vi "Concatenate_Blocks.vi"() -> (5 "Plug in titles":string[](array[string]), 7 "Plug in values":string[](array[string]))   [LabVIEW 2012]
uses:
  Controls/Post_Process.ctl
  Controls/Graph_Type.ctl
  Globals/Meas_global.vi
  <vilib>/Analysis/NI_AALBase.lvlib
panel:
  in  "PDF":bool=TRUE
  out "No Of Spectral Averages":i32
  out "Autocorrelation":cluster{dbl, dbl, dbl[]}[](graph)
  in  "Show Smooth":bool=TRUE
  in  "Save Plots":bool
  in  "No of averged samples in spectra":i32=4096
  in  "Calculate Spectra and Histogram?":bool
  out "Spectra":cluster{dbl, dbl, dbl[]}[](graph)
  in  "Averaging samples":i32=5 min=1 max=1000
  out "Histogram/Pdf":T1(graph)
  out "Waveform Graph":dbl[][](graph)
  in  "Channels to Plot":i32[](array[ring])=[0] items=["FF (C)", "Save Nothing"]
  # "Run this VI to update the channel names"
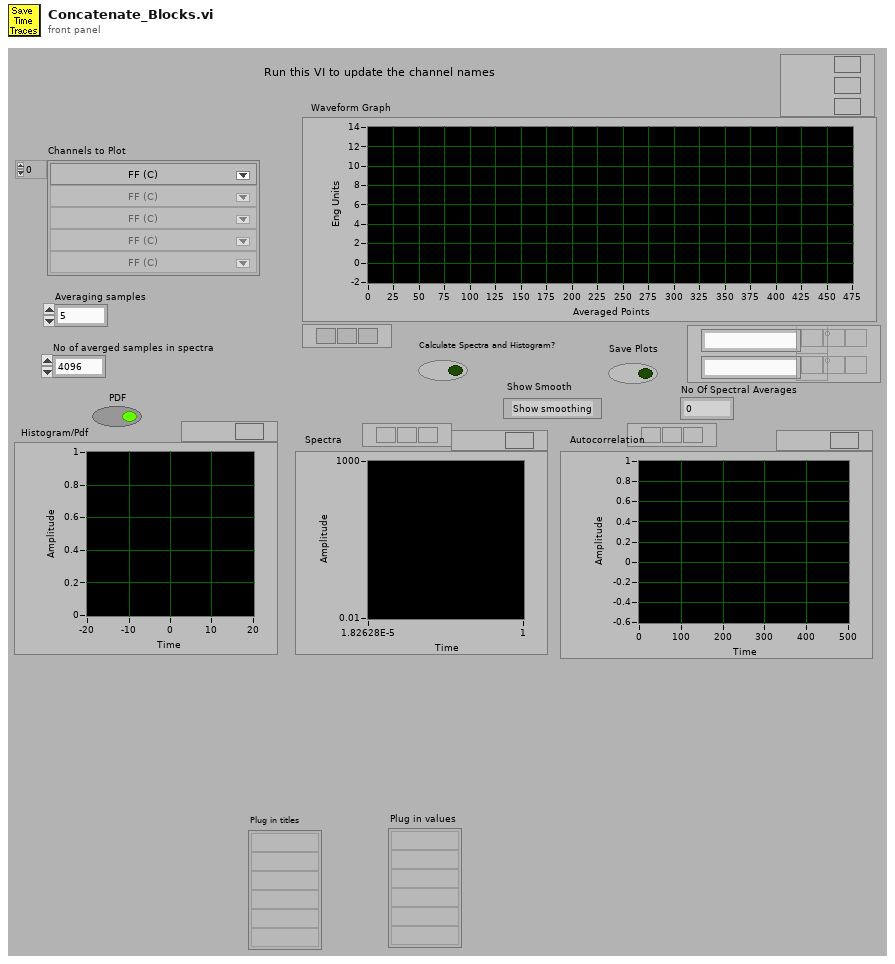
[diagram p1: front panel]
types:
  T1 = cluster{"element":dbl, dbl, "1D histogram or PDF":dbl[]}[]
  T2 = typedef "Analysis_info_cluster.ctl" = cluster{"Colour":u32, "Inst type":T3, "Inst name":string, "Symbol":string, "Code name":string, "Extra Info":string, "Inst Array":T4, "Extra Titles":string[], "Extra Values":string[], "U":dbl, "u^2":dbl, "u^3":dbl, "u^4":dbl, "Skew_u":dbl, "Kurt_u":dbl, "Sd Error in Mean":dbl, "% u'/U":dbl, "X":dbl, "Y":dbl, "Z":dbl, "Timescale integral to 25%":dbl, "Sd Error in Variance":dbl, "Calib File":path, "Calib Constants":dbl[], "Output Position":bool, "Full Stats":bool, "Av Sampling Rate":dbl, "Av No of Samples":dbl, "Total Meas Time (s)":dbl, "ADAM Ch Name":string}
  T3 = typedef "Inst_type.ctl" = enum16{"Propeller anemometer", "Raw voltage", "Pressure Transducer", "Pitot-static tube", "Preston tube", "Hot wire", "Cross wire 1", "Cross wire 2", "Generic Linear", "Generic Polynomial", "Generic BackPoly", "Fast FID", "Thermocouple", "Cold wire", "Pulsed Wire", "LDA Vel", "LDA Tran time", "LDA Arr time"}
  T4 = typedef "Instrument_Array.ctl" = enum16{"PWA", "LDA", "Analogue"}
  T5 = typedef "Time_Trace_Cluster.ctl" = cluster{"Weighting":dbl[], "Time (s)":dbl[], "Voltage":dbl[], "Eng Values":dbl[]}
  T6 = typedef "Post_Process.ctl" = enum16{"Take New Data", "Post Process Raw Data File"}
  T7 = typedef "Graph_Type.ctl" = enum16{"Show no graph", "Voltage trace", "Velocity trace", "Vel histogram", "Spectrum", "f.E(f) v Log f", "Auto-Corr"}
  T8 = cluster{"Plot 1":u16, "Plot 2":u16, "Save graph":u16, "Plot Type":T7}
  T9 = cluster{"element":dbl, dbl, "1D histogram or PDF":dbl[]}
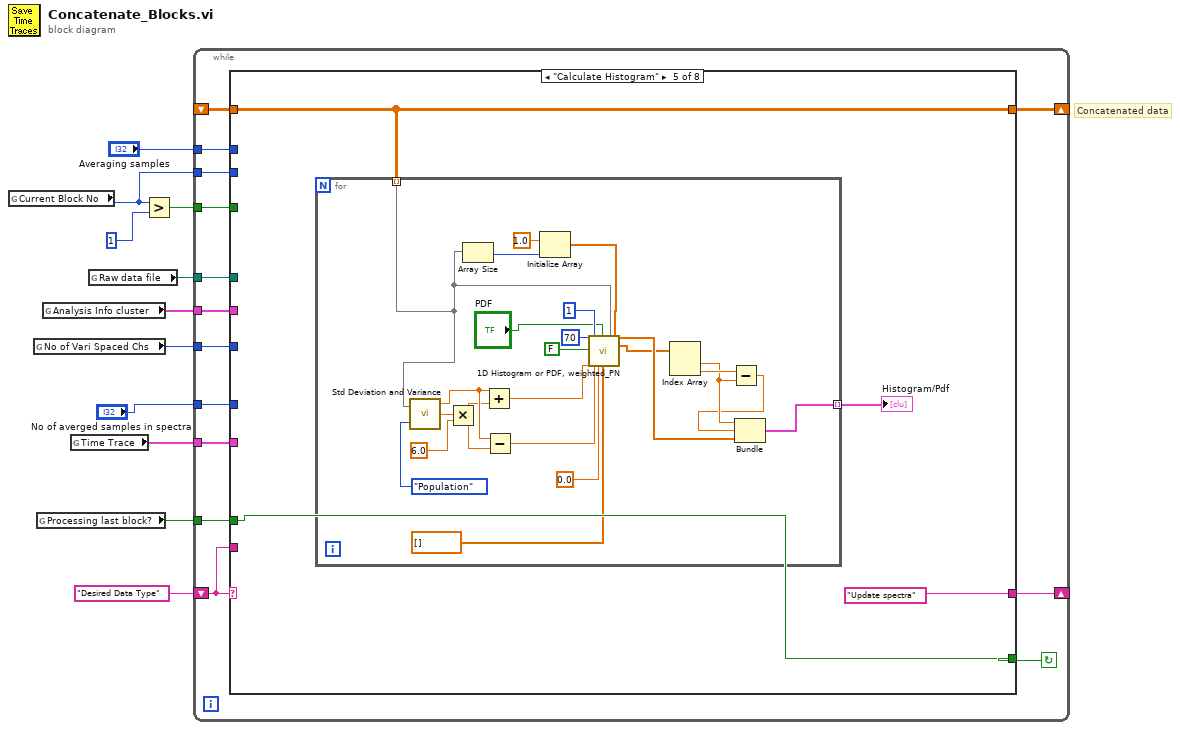
[diagram p0: block diagram]
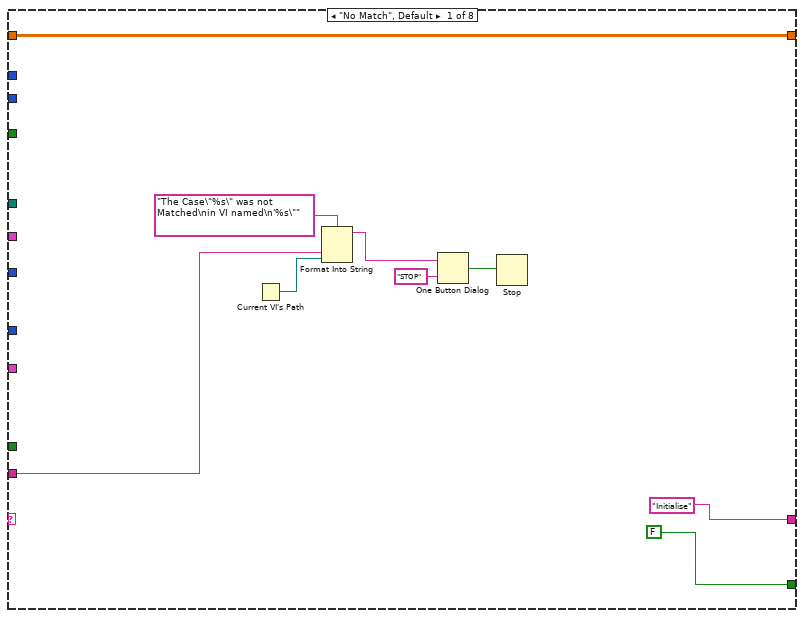
[diagram p2: hidden frame]
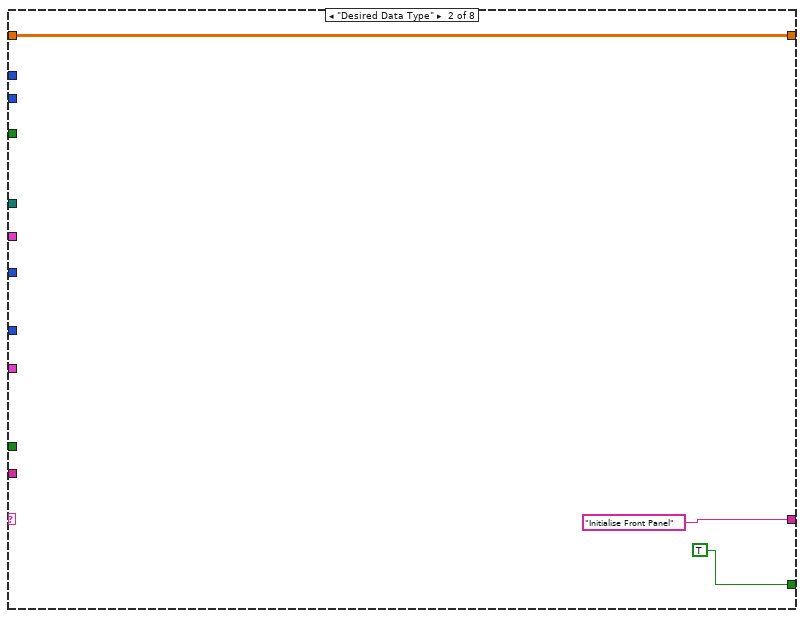
[diagram p3: hidden frame]
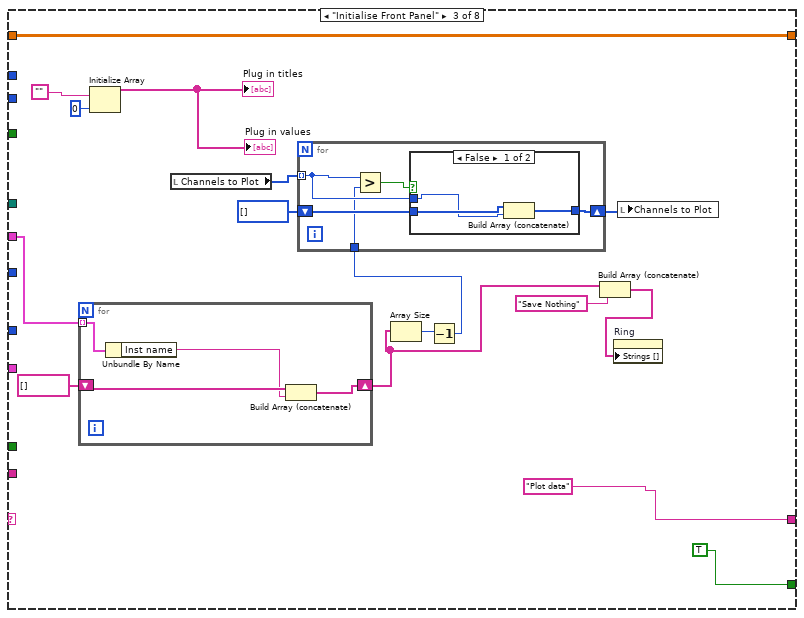
[diagram p4: hidden frame]
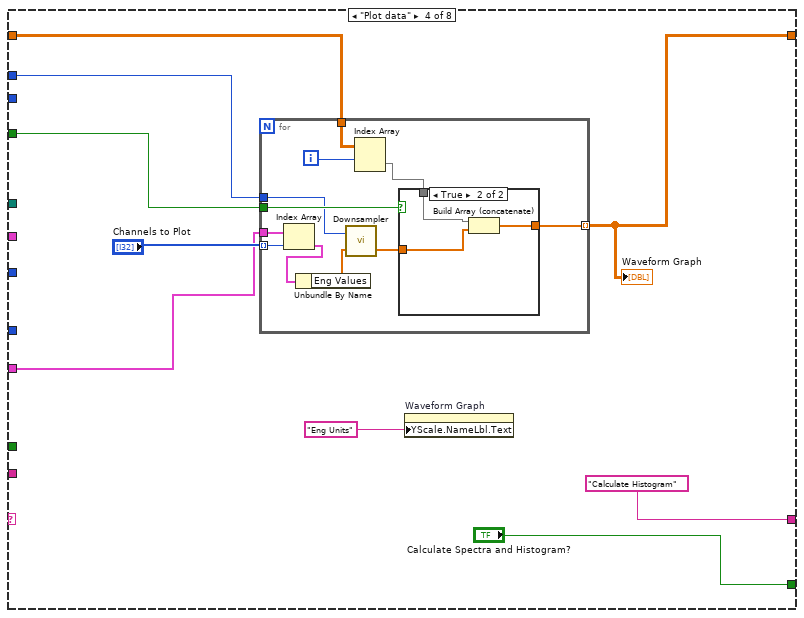
[diagram p6: hidden frame]
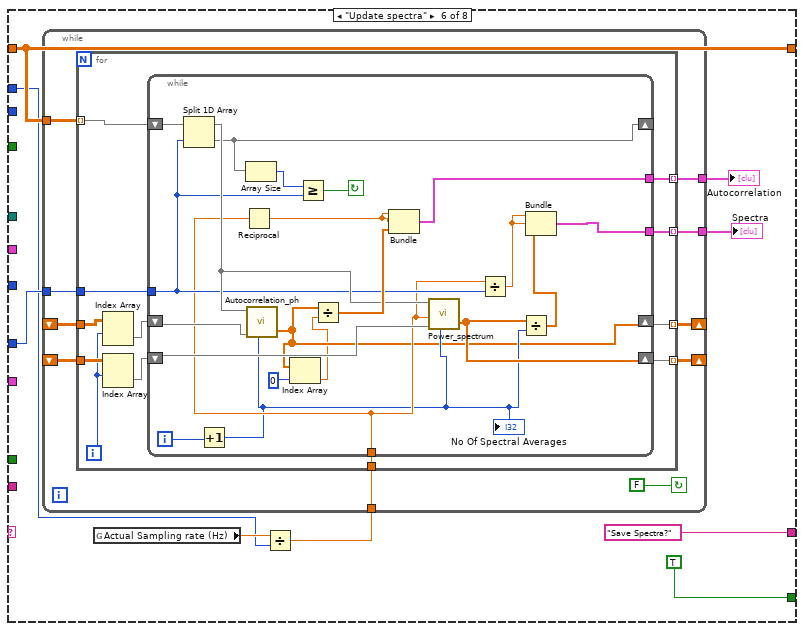
[diagram p8: hidden frame]
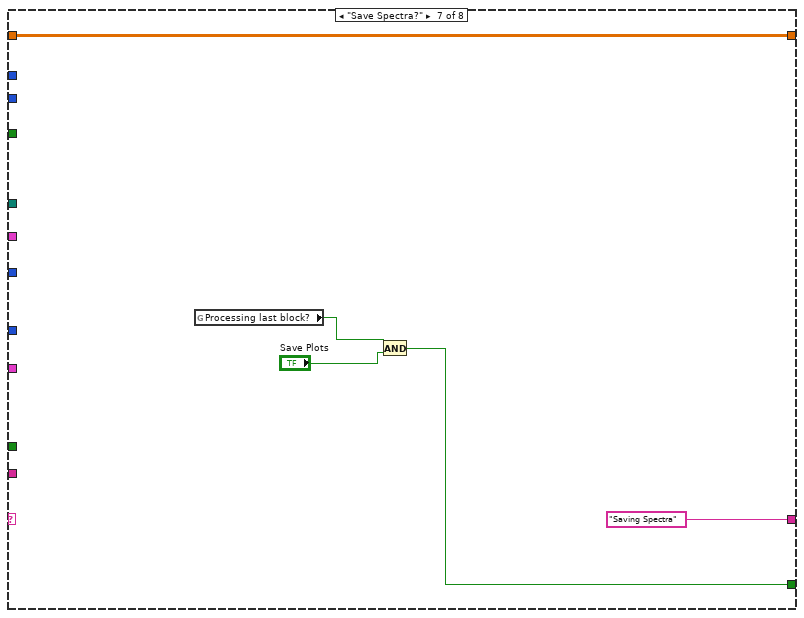
[diagram p9: hidden frame]
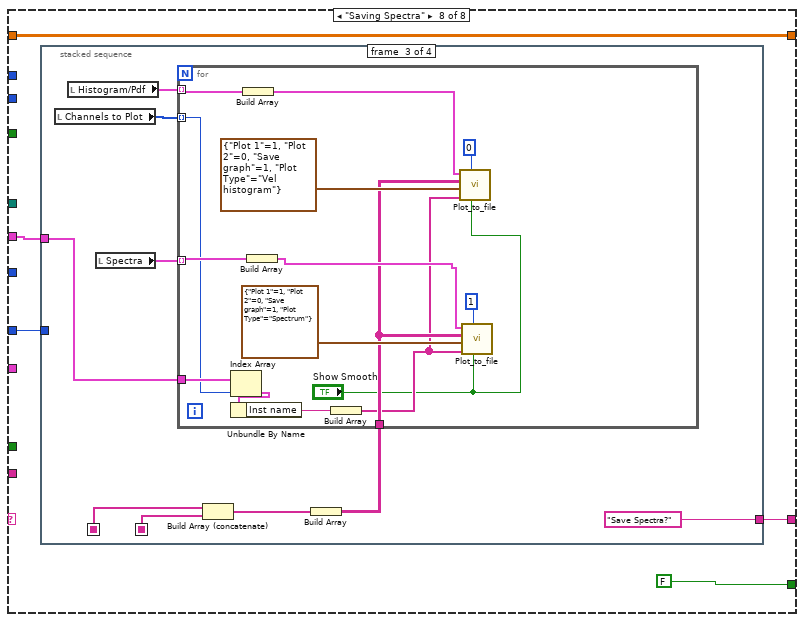
[diagram p10: hidden frame]
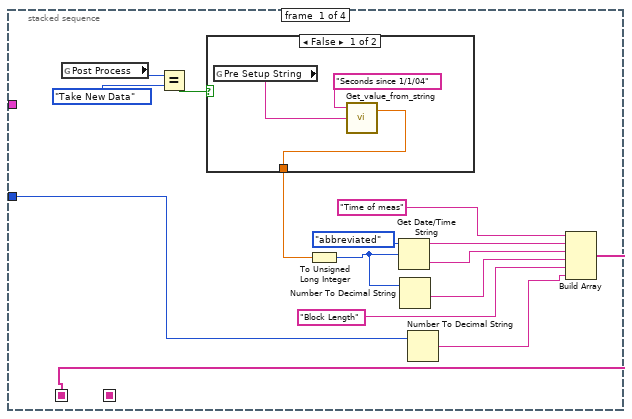
[diagram p11: hidden frame]
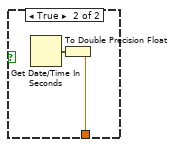
[diagram p12: hidden frame]
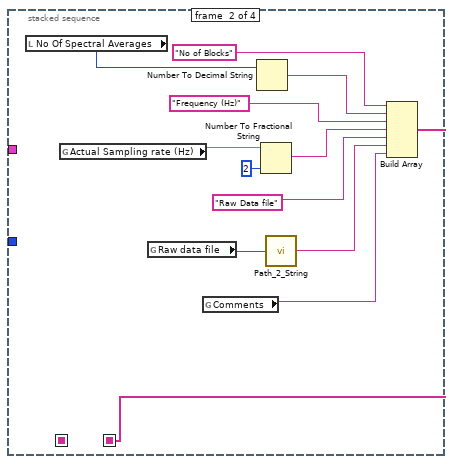
[diagram p13: hidden frame]
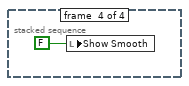
[diagram p14: hidden frame]
diagram:
  # "Concatenated data"
  n1 = global read "Meas_global.vi" "Current Block No"() -> (w8:i32)
  n2 = global read "Meas_global.vi" "No of Vari Spaced Chs"() -> (w6:i32)
  n3 = global read "Meas_global.vi" "Processing last block?"() -> (w1:bool)
  n4 = global read "Meas_global.vi" "Analysis Info cluster"() -> (w7:T2[])
  n5 = global read "Meas_global.vi" "Time Trace"() -> (w3:T5[])
  n6 = global read "Meas_global.vi" "Raw data file"() -> (w10:path)
  n7 = Greater?(x=w8, y=1) -> (0:w5:bool)
  n8 = while {
    shift-left: "Desired Data Type" -> [w23]
    shift-right: [w24] -> _
    tunnel: w10 -> [w22]
    tunnel: w5 -> [w21]
    tunnel: w8 -> [w20]
    tunnel: w7 -> [w19]
    tunnel: w6 -> [w18]
    shift-right: [w16] -> _
    shift-left: _ -> [w17]
    tunnel: "No of averged samples in spectra" -> [w15]
    tunnel: w3 -> [w14]
    tunnel: "Averaging samples" -> [w13]
    tunnel: w1 -> [w12]
    stop <- w25 continue-if-true
    n9 = case shown="\"Calculate Histogram\"" w23 {
      tunnel: [FALSE TRUE TRUE "Calculate Spectra and Histogram?" w92 TRUE ("Calculate Spectra and Histogram?") w170 FALSE ("Calculate Spectra and Histogram?")] -> w25
      tunnel: ["Initialise" "Initialise Front Panel" "Plot data" "Calculate Histogram" ("t") "Update spectra" "Save Spectra?" "Saving Spectra" w178] -> w24
      tunnel: w23 -> [w29 _ _ _ _ _ _ _]
      tunnel: w22 -> [_ _ _ _ _ _ _ _]
      tunnel: w21 -> [_ _ _ w74 _ _ _ _]
      tunnel: w20 -> [_ _ _ _ _ _ _ _]
      tunnel: w19 -> [_ _ w40 _ _ _ _ w177]
      tunnel: w18 -> [_ _ _ _ _ _ _ _]
      tunnel: w17 -> [w26 w35 w43 w75 w94 w123 w174 w179]
      tunnel: [w26 w35 w43 w72 w94 w123 w174 w179] -> w16
      tunnel: w15 -> [_ _ _ _ _ w124 _ w175]
      tunnel: w14 -> [_ _ _ w68 _ _ _ _]
      tunnel: w13 -> [_ _ _ w67 _ w121 _ _]
      tunnel: w12 -> [_ _ _ _ w92 _ _ _]
      frame "No Match", Default {
        n10 = Current VI's Path() -> (path=w28:path)
        n11 = Format Into String(format string="The Case\"%s\" was not Matched\nin VI named\n'%s\"" ("Format String"), w29, w28) -> (resulting string=w32:string)  [unwired: 2 in, 1 out]
        n12 = One Button Dialog(message=w32, button name ("OK")="STOP") -> (true=w30:bool)
        n13 = Stop(stop? (T)=w30) -> ()
      }
      frame "Desired Data Type" {
      }
      frame "Initialise Front Panel" {
        n14 = for {
          tunnel: w40 -> [w57] mode=indexing
          shift-right: [w55] -> w39
          shift-left: string[] [] -> [w56]
          n15 = Unbundle By Name(w57) -> ("Inst name"=w54:string)
          n16 = Build Array (concatenate)(w56, w54) -> (w55:string[])
        }
        n17 = Initialize Array("", 0) -> (→"Plug in values" →"Plug in titles":string[])
        n18 = local read "Channels to Plot"() -> (w50:i32[])
        n19 = Array Size(array=w39) -> (size(s)=w45:i32)
        n20 = Decrement(x=w45) -> (x-1=w44:i32)
        n21 = for {
          tunnel: w50 -> [w59] mode=indexing
          shift-right: [w60] -> w48
          shift-left: i32[] [] -> [w61]
          tunnel: w44 -> [w58]
          n22 = Greater?(x=w59, y=w58) -> (0:w62:bool)
          n23 = case shown="False" w62 {
            tunnel: w61 -> [w65 w66]
            tunnel: [w64 w66] -> w60
            tunnel: w59 -> [w63 _]
            frame False {
              n24 = Build Array (concatenate)(w65, w63) -> (w64:i32[])
            }
            frame True {
            }
          }
        }
        n25 = Build Array (concatenate)(w39, "Save Nothing") -> (w46:string[])
        n26 = property on="Ring" class="Ring (strict)"("Strings []"=w46) -> ()  [unwired: 2 in, 2 out]
        n27 = local write "Channels to Plot"(w48) -> ()
      }
      frame "Plot data" {
        n28 = for {
          tunnel: w68 -> [w86]
          tunnel: "Channels to Plot" -> [w85] mode=indexing
          tunnel: w75 -> [w82]
          tunnel: [w83] -> w72 mode=indexing
          tunnel: w74 -> [w84]
          tunnel: w67 -> [w76]
          i -> [w81]
          n29 = Index Array(array=w86, index=w85) -> (element=w78:T5)
          n30 = Unbundle By Name(w78) -> ("Eng Values"=w77:dbl[])
          n31 = call "Downsampler.vi"("Input Array"=w77, "Averaging samples"=w76) -> ("Downsampled Array"=w79:dbl[])  [unwired: 1 out]
          n32 = Index Array(array=w82, index (row)=w81) -> (element=w80:dbl[])  [unwired: 1 in]
          n33 = case shown="True" w84 {
            tunnel: w80 -> [_ w90]
            tunnel: w79 -> [w87 w89]
            tunnel: [w87 w88] -> w83
            frame False {
            }
            frame True {
              n34 = Build Array (concatenate)(w90, w89) -> (w88:dbl[])
            }
          }
        }
        "Waveform Graph" <- w72
        n35 = property on="Waveform Graph" class="WFGraph (strict)"("YScale.NameLbl.Text"="Eng Units") -> ()  [unwired: 2 in, 2 out]
      }
      frame "Calculate Histogram" {
        n36 = for {
          tunnel: w94 -> [w95] mode=indexing
          tunnel: [w96] -> w91 mode=indexing
          n37 = call <vilib>:"Std Deviation and Variance.vi"("X"=w95, "Weighting (Sample)"=enum16{"Sample", "Population"}."Population") -> ("mean"=w110:dbl, "standard deviation"=w109:dbl)  [unwired: 1 out]
          n38 = Multiply(x=w109, y=6.0) -> (x*y=w107:dbl)
          n39 = Array Size(array=w95) -> (size(s)=w114:i32)
          n40 = Add(x=w110, y=w107) -> (x+y=w105:dbl)
          n41 = Subtract(x=w110, y=w107) -> (x-y=w104:dbl)
          n42 = Initialize Array(1.0 ("element"), w114) -> (w112:dbl[])
          n43 = call "1D Histogram or PDF, weighted_PN.vi"("Nbins"=70, "Mean shift"=FALSE, "max"=w105, "Current block no."=1, "min"=w104, "Shift SumW in"=0.0, "PDF"="PDF", "Shift PDF in"=dbl[] [], "1D data"=w95, "Weights"=w112) -> ("1D histogram or PDF"=w111:dbl[], "bin centre vals."=w100:dbl[])  [unwired: 13 in, 3 out]
          n44 = Index Array(array=w100) -> (element #1=w98:dbl, element #2=w99:dbl)  [unwired: 2 in]
          n45 = Subtract(x=w99, y=w98) -> (x-y=w97:dbl)
          n46 = Bundle("element"=w98, w97, "1D histogram or PDF"=w111) -> (w96:T9)  [unwired: 1 out]
        }
        "Histogram/Pdf" <- w91
      }
      frame "Update spectra" {
        n47 = global read "Meas_global.vi" "Actual Sampling rate (Hz)"() -> (w122:dbl)
        n48 = Divide(x=w122, y=w121) -> (x/y=w120:dbl)
        n49 = while {
          shift-left: _ -> [w133]
          shift-right: [w136] -> _
          tunnel: w124 -> [w134]
          shift-right: [w131] -> _
          shift-left: _ -> [w132]
          tunnel: w123 -> [w130]
          tunnel: w120 -> [w129]
          tunnel: [w128] -> w119
          tunnel: [w127] -> w118
          stop <- FALSE continue-if-true
          n50 = for {
            tunnel: [w145] -> w136 mode=indexing
            tunnel: w134 -> [w148]
            tunnel: w133 -> [w141]
            tunnel: w132 -> [w143]
            tunnel: [w146] -> w131 mode=indexing
            tunnel: w130 -> [w147] mode=indexing
            tunnel: w129 -> [w144]
            tunnel: [w138] -> w128 mode=indexing
            tunnel: [w137] -> w127 mode=indexing
            i -> [w139]
            n51 = Index Array(array=w143, index (row)=w139) -> (element=w142:dbl[])  [unwired: 1 in]
            n52 = Index Array(array=w141, index (row)=w139) -> (element=w140:dbl[])  [unwired: 1 in]
            n53 = while {
              tunnel: w148 -> [w160]
              shift-right: [w154] -> _
              shift-left: w147 -> [w157]
              shift-right: [w165] -> w145
              shift-left: w140 -> [w163]
              shift-right: [w150] -> w146
              shift-left: w142 -> [w164]
              tunnel: w144 -> [w158]
              tunnel: [w156] -> w138
              tunnel: [w155] -> w137
              i -> [w153]
              stop <- w159 continue-if-true
              n54 = Split 1D Array(array=w157, index=w160) -> (first subarray=w162:dbl[], second subarray=w154:dbl[])
              n55 = Increment(x=w153) -> (x+1=w152:i32)
              "No Of Spectral Averages" <- w152
              n56 = Reciprocal(x=w158) -> (1/x=w167:dbl)
              n57 = Array Size(array=w154) -> (size(s)=w161:i32)
              n58 = call "Autocorrelation_ph.vi"("X"=w162, "Autocorrelation of X"=w164, "Block No"=w152) -> ("Autocorrelation of X"=w150:dbl[])  [unwired: 3 in]
              n59 = Index Array(array=w150, index=0 ("Index")) -> (element=w149:dbl)
              n60 = Greater Or Equal?(x=w161, y=w160) -> (x >= y?=w159:bool)
              n61 = Divide(x=w150, y=w149) -> (x/y=w166:dbl[])
              n62 = Bundle(w167, w167, w166) -> (w156:cluster{dbl, dbl, dbl[]})  [unwired: 1 out]
              n63 = call "Power_spectrum.vi"("U"=w162, "Sampling frequency"=w158, "Spectrum input array"=w163, "Block No"=w152) -> ("Spectrum output array"=w165:dbl[])  [unwired: 1 in, 1 out]
              n64 = Divide(x=w158, y=w160) -> (x/y=w169:dbl)
              n65 = Divide(x=w165, y=w152) -> (x/y=w168:dbl[])
              n66 = Bundle(w169, w169, w168) -> (w155:cluster{dbl, dbl, dbl[]})  [unwired: 1 out]
            }
          }
        }
        "Spectra" <- w118
        "Autocorrelation" <- w119
      }
      frame "Save Spectra?" {
        n67 = global read "Meas_global.vi" "Processing last block?"() -> (w171:bool)
        n68 = And(x=w171, y="Save Plots") -> (x .and. y?=w170:bool)
      }
      frame "Saving Spectra" {
        n69 = stacked-sequence {
          seq-local: [w183 _ _ _] -> [_ _ w218 _]
          seq-local: [_ w202 _ _] -> [_ _ w217 _]
          tunnel: [_ _ "Save Spectra?" _] -> w178
          tunnel: w177 -> [_ _ w212 _]
          tunnel: w175 -> [w181 _ _ _]
          frame #0 {
            n70 = global read "Meas_global.vi" "Post Process"() -> (w185:T6)
            n71 = Equal?(x=w185, y=Post_Process."Take New Data" ("Post Process")) -> (x = y?=w186:bool)
            n72 = case shown="False" w186 {
              tunnel: [w194 w198] -> w187
              frame False {
                n73 = global read "Meas_global.vi" "Pre Setup String"() -> (w195:string)
                n74 = call "Get_value_from_string.vi"("Input string"=w195, "Variable name"="Seconds since 1/1/04") -> ("Value"=w194:dbl)  [unwired: 1 in, 1 out]
              }
              frame True {
                n75 = Get Date/Time In Seconds() -> (seconds since 1Jan1904=w197:timestamp)
                n76 = To Double Precision Float(number=w197) -> (double precision float=w198:dbl)
              }
            }
            n77 = To Unsigned Long Integer(number=w187) -> (unsigned 32bit integer=w191:u32)
            n78 = Get Date/Time String(date format (0)=enum16{"short", "long", "abbreviated"}."abbreviated", seconds (now)=w191) -> (date string=w189:string, time string=w190:string)  [unwired: 1 out]
            n79 = Number To Decimal String(number=w191) -> (decimal integer string=w192:string)  [unwired: 1 out]
            n80 = Number To Decimal String(number=w181) -> (decimal integer string=w180:string)  [unwired: 1 out]
            n81 = Build Array("Time of meas", w189, w190, w192, "Block Length" ("element"), w180) -> (w183:string[])
          }
          frame #1 {
            n82 = local read "No Of Spectral Averages"() -> (w199:i32)
            n83 = global read "Meas_global.vi" "Actual Sampling rate (Hz)"() -> (w203:dbl)
            n84 = global read "Meas_global.vi" "Raw data file"() -> (w209:path)
            n85 = global read "Meas_global.vi" "Comments"() -> (w208:string)
            n86 = Number To Decimal String(number=w199) -> (decimal integer string=w200:string)  [unwired: 1 out]
            n87 = Number To Fractional String(number=w203, precision (6)=i16 2) -> (F-format string=w206:string)  [unwired: 2 out]
            n88 = call "Path_2_String.vi"("Real Path"=w209) -> ("Path String"=w210:string)
            n89 = Build Array("No of Blocks", w200, "Frequency (Hz)", w206, "Raw Data file", w210, w208) -> (w202:string[])
          }
          frame #2 {
            n90 = local read "Channels to Plot"() -> (w211:i32[])
            n91 = local read "Histogram/Pdf"() -> (w213:T1)
            n92 = local read "Spectra"() -> (w214:cluster{dbl, dbl, dbl[]}[])
            n93 = Build Array (concatenate)(w218, w217) -> (w216:string[])
            n94 = Build Array(w216) -> (w215:string[][])
            n95 = for {
              tunnel: w215 -> [w223]
              tunnel: w214 -> [w229] mode=indexing
              tunnel: w213 -> [w231] mode=indexing
              tunnel: w212 -> [w227]
              tunnel: w211 -> [w226] mode=indexing
              n96 = Index Array(array=w227, index=w226) -> (element=w224:T2)
              n97 = Unbundle By Name(w224) -> ("Inst name"=w225:string)
              n98 = Build Array(w231) -> (w230:T1)
              n99 = Build Array(w229) -> (w228:cluster{dbl, dbl, dbl[]}[])
              n100 = Build Array(w225) -> (w222:string[])
              n101 = call "Plot_to_file.vi"("Show Smooth"="Show Smooth", "Start trace No"=0, "Trace names"=w222, "Graph"=T8 {"Plot 1"=1, "Plot 2"=0, "Save graph"=1, "Plot Type"=enum."Vel histogram"}, "Plot file label"=w223, "Plot data"=w230) -> ()  [unwired: 6 out]
              n102 = call "Plot_to_file.vi"("Show Smooth"="Show Smooth", "Start trace No"=1, "Trace names"=w222, "Graph"=T8 {"Plot 1"=1, "Plot 2"=0, "Save graph"=1, "Plot Type"=enum."Spectrum"}, "Plot file label"=w223, "Plot data"=w228) -> ()  [unwired: 6 out]
            }
          }
          frame #3 {
            n103 = local write "Show Smooth"(FALSE ("Show Smooth")) -> ()
          }
        }
      }
    }
  }
